vi "Set Color.vi"(9 "index":i32, 11 "list in":T1[](array[typedef]) {"Creation Date" format="%<%x>T"; "Last Updated" format="%<%x>T"}) -> (3 "list out":T1[](array[typedef]) {"Creation Date" format="%<%x>T"; "Last Updated" format="%<%x>T"})   [LabVIEW 2018]
uses:
  Type Defs/SR Cluster.ctl
  Type Defs/SR Status.ctl
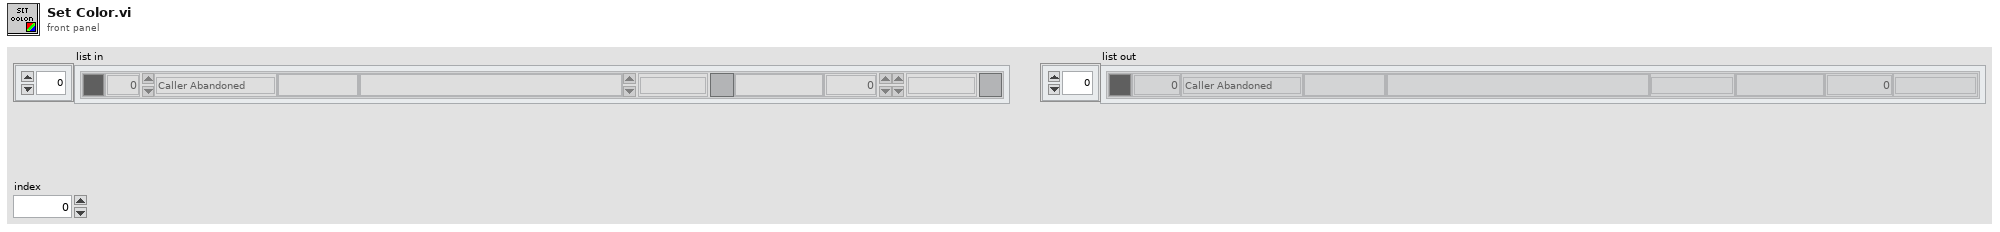
[diagram p1: front panel]
types:
  T1 = typedef "SR Cluster.ctl" = cluster{"Color":u32, "SR Number":i32, "SR Status":T2, "SR Type":string, "Summary":string, "Last Updated":timestamp, "Service Level":string, "Days Open":dbl, "Creation Date":timestamp}
  T2 = typedef "SR Status.ctl" = enum16{"Caller Abandoned", "Created in Error", "Expired", "Forum Resolved AE", "Forum Resolved Customer", "IN WORK", "IN WORK Collab with AES", "IN WORK Collab with PSE", "IN WORK Collab with SE", "IN WORK Customer Added Note", "IN WORK Escalation", "IN WORK Wait on Customer", "Open", "Potentially Resolved", "Presumed Resolved", "RMA Approved for Return", "Resolved", "Passed Off"}
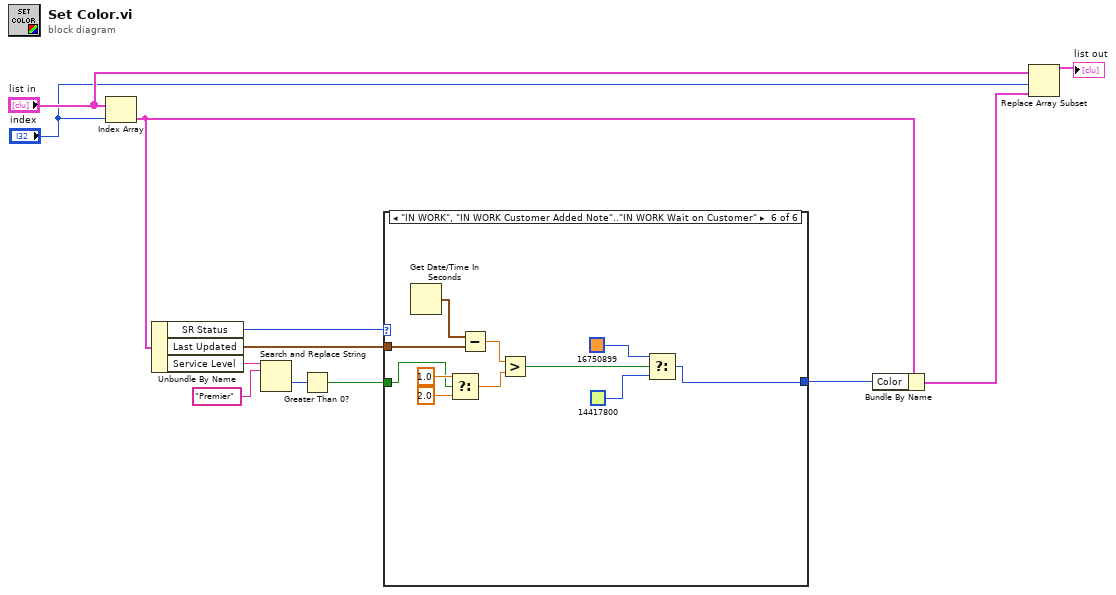
[diagram p0: block diagram]
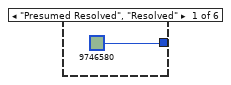
[diagram p2: hidden frame]
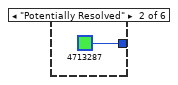
[diagram p3: hidden frame]
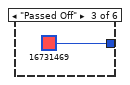
[diagram p4: hidden frame]
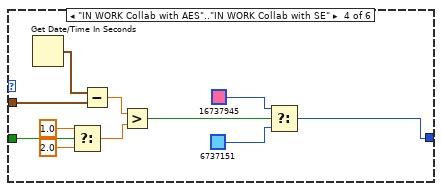
[diagram p5: hidden frame]
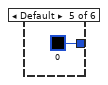
[diagram p6: hidden frame]
diagram:
  n1 = Index Array(array="list in", index="index") -> (element=w3:T1)
  n2 = Unbundle By Name(w3) -> ("SR Status"=w7:T2, "Last Updated"=w5:timestamp, "Service Level"=w10:string)
  n3 = Search and Replace String(input string=w10, search string="Premier") -> (offset past replacement=w8:i32)  [unwired: 6 in, 3 out]
  n4 = Greater Than 0?(x=w8) -> (x > 0?=w6:bool)
  n5 = case shown="\"IN WORK\", \"IN WORK Customer Added Note\"..\"IN WORK Wait on Customer\"" w7 {
    tunnel: w6 -> [_ _ _ w26 _ w30]
    tunnel: w5 -> [_ _ _ w23 _ w29]
    tunnel: [u32 9746580 u32 4713287 u32 16731469 w16 u32 0 w28] -> w4
    frame "Presumed Resolved", "Resolved" {
    }
    frame "Potentially Resolved" {
    }
    frame "Passed Off" {
    }
    frame "IN WORK Collab with AES".."IN WORK Collab with SE" {
      n6 = Get Date/Time In Seconds() -> (seconds since 1Jan1904=w22:timestamp)
      n7 = Select(t=1.0, s=w26, f=2.0) -> (s? t:f=w20:dbl)
      n8 = Subtract(x=w22, y=w23) -> (x-y=w21:dbl)
      n9 = Greater?(x=w21, y=w20) -> (0:w17:bool)
      n10 = Select(t=u32 16737945, s=w17, f=u32 6737151) -> (s? t:f=w16:u32)
    }
    frame Default {
    }
    frame "IN WORK", "IN WORK Customer Added Note".."IN WORK Wait on Customer" {
      n11 = Get Date/Time In Seconds() -> (seconds since 1Jan1904=w35:timestamp)
      n12 = Select(t=1.0, s=w30, f=2.0) -> (s? t:f=w37:dbl)
      n13 = Subtract(x=w35, y=w29) -> (x-y=w36:dbl)
      n14 = Greater?(x=w36, y=w37) -> (0:w38:bool)
      n15 = Select(t=u32 16750899, s=w38, f=u32 14417800) -> (s? t:f=w28:u32)
    }
  }
  n16 = Bundle By Name(cluster=w3, "Color"=w4) -> (w12:T1)
  n17 = Replace Array Subset(array="list in", new element=w12, index="index") -> (→"list out":T1[])
